vi "Acq Fetch Waveform (I16 Data Ref) - Timeout fix.vi"(0 "session in":refnum<class "Digitizer Control.lvclass">, 2 "elements to read":u32, 5 "error in (no error)":errorcluster, 7 "timeout (ms)":i32=5000, 8 "channel index":i32, 9 "clear time out error? (F)":bool) -> (13 "timed out?":bool, 14 "session out":refnum<class "Digitizer Control.lvclass">, 15 "sample data":refnum<data-value>, 16 "elements in region":u32, 17 "elements remaining":u32, 19 "error out":errorcluster)   [LabVIEW 2021, in "Digitizer Control.lvclass"]
doc: "This VI returns a reference to the host DMA buffer part containing the requested amount of acquired sample data as an array of I16s. Use the <B>Acq Configure Channel.vi</B> to configure the channel parameters, the <B>Acq Configure Transfer.vi</B> to configure the waveform transfer, and the <B>Acq Configure Start Trigger.vi</B> to configure the start trigger, then use the <B>Acq Initiate.vi</B> to initiate the acquisition. After the acquisition is initiated, use this VI to fetch the acquired sample data. Use the <B>Acq Get Status.vi</B> to check the acquisition status and the <B>Acq Stop.vi</B> to stop an acquisition.\n\nInputs:\n\n<B>session in</B>: The device session.\n\n<B>channel index</B>: The index of the channel to read.\n\n<B>elements to read</B>: The desired number of I16 elements the referenced array should contain. The actual number of elements is returned on the <B>elements in region</B> output.\n\n<B>timeout</B>: The maximum amount of time, in milliseconds, this VI is allowed to wait for the requested number of elements to become available.\n\n<B>clear time out error?</B>: If this input is true, then the <B>error out</B> output does not return the time out error.\n\nOutputs:\n\n<B>session out</B>: The device session passed on the <B>session in</B> input.\n\n<B>sample data</B>: Reference to an array of I16s containing the acquired sample data. The samples are using fixed point representation: the size of a sample is <B>sample size (bits)</B> bits. The bits of the samples are placed in the I16 elements with LSB first bit packing. To convert the returned I16 array to samples scaled to Volts: unpack the samples then multiply the samples by <B>sample scale factor</B> * 2^-( <B>sample size (bits)</B> ), where <B>sample scale factor</B> is returned by the <B>Acq Configure Channel.vi</B>, while <B>sample size (bits)</B> is returned by the <B>Acq Configure Transfer.vi</B>. The size of the array referenced by this output is returned on the <B>elements in region</B> output. NOTE: The returned data value reference must be deleted after it is no longer needed.\n\n<B>elements in region</B>: The number of I16 elements available in the array referenced by the <B>sample data</B> output.\n\n<B>elements remaining</B>: The number of additional elements remaining in the host DMA buffer that are available for reading.\n\n<B>timed out?</B>: A true on this output indicates that the fetch operation timed out.\n\nNotes:\n\nDo not mix the different Acq Fetch Waveform VIs. Once this VI is called on a channel, use only this VI to fetch the acquired samples on that channel. If you want to use another fetch VI, then it is recommended to reconfigure the transfer first using the <B>Acq Configure Transfer.vi</B>."
uses:
  Digitizer Control.lvclass
  Digitizer Control.lvclass/Digitizer Control.ctl
  <vilib>/rvi/errors/niLvFpgaAdjustHostInterfaceError.vi
  <vilib>/rvi/interface/nirviMethod/nirviMethod.xnode
  <vilib>/ErrorRing/Error Ring.xnode
  <vilib>/FPGAPlugInAG/Dynamic/niLvFpga_AcquireReadRegionFifo_Dynamic.vi
  <vilib>/rvi/errors/niLvFpgaMergeErrorWithErrorCode.vi
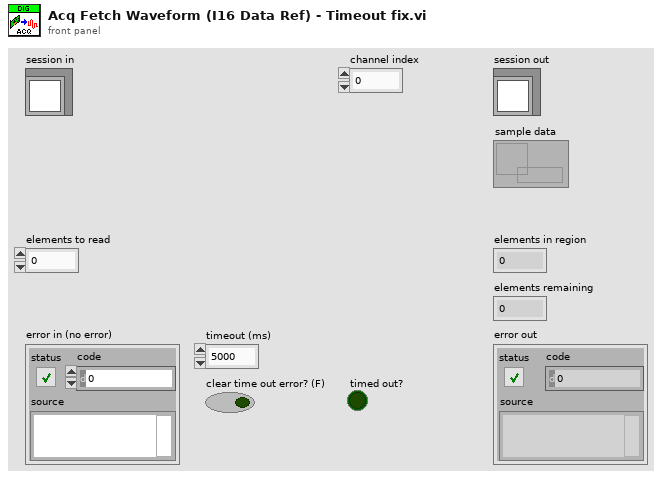
[diagram p1: front panel]
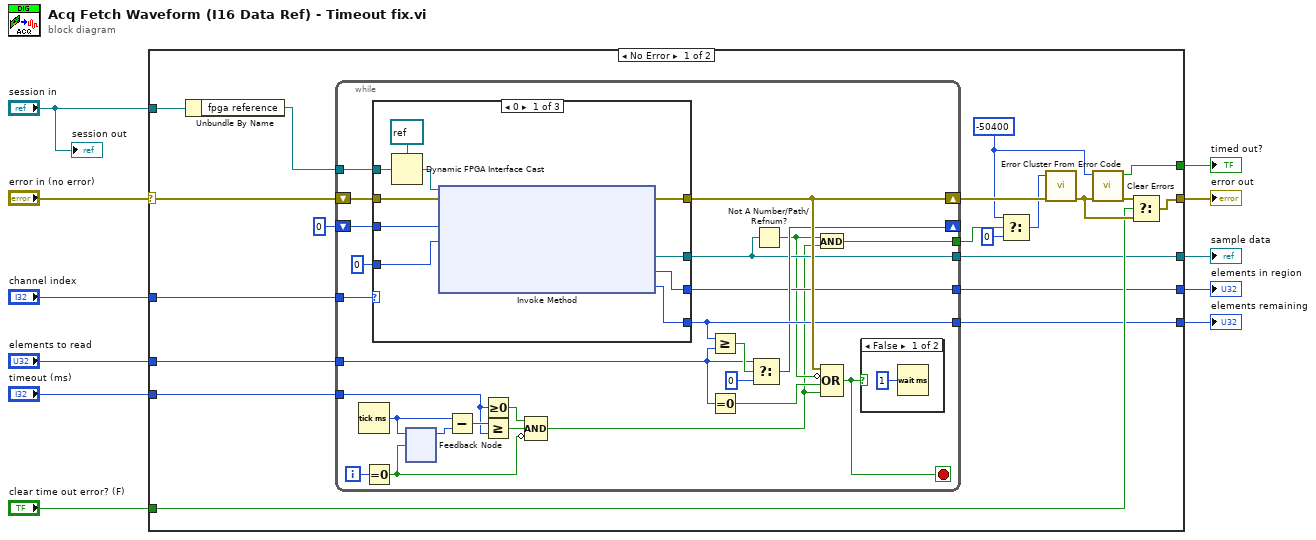
[diagram p0: block diagram]
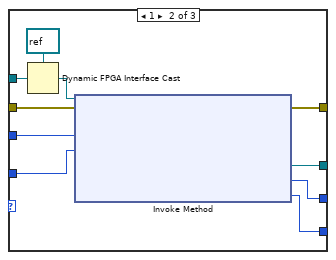
[diagram p3: hidden frame]
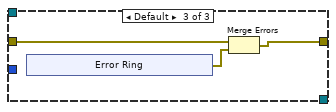
[diagram p4: hidden frame]
diagram:
  n1 = case shown="No Error" "error in (no error)" {
    selector: "error in (no error)" -> [w22 w87]
    tunnel: "elements to read" -> [w17 _]
    tunnel: [w30 w87] -> w4
    tunnel: "timeout (ms)" -> [w16 _]
    tunnel: "session in" -> [w26 _]
    tunnel: [w24 _] -> w8
    tunnel: [w25 _] -> w6
    tunnel: [w23 _] -> w5
    tunnel: "clear time out error? (F)" -> [w27 _]
    tunnel: [w20 _] -> w2
    tunnel: "channel index" -> [w19 _]
    frame No Error {
      w14 = -50400 ("specific error code to clear (0: all)")
      n2 = Unbundle By Name(w26) -> ("fpga reference"=w21:refnum<k20>)
      n3 = while {
        tunnel: [w38] -> w25
        tunnel: [w50] -> w24
        tunnel: [w39] -> w23
        tunnel: w21 -> [w54]
        tunnel: w19 -> [w53]
        shift-right: [w57] -> w29
        shift-left: w22 -> [w55]
        shift-right: [w47] -> _
        shift-left: u32 0 -> [w52]
        tunnel: w17 -> [w37]
        tunnel: w16 -> [w41]
        tunnel: [w32] -> w15
        i -> [w36]
        stop <- w35 stop-if-true
        n4 = Tick Count (ms)() -> (millisecond timer value=w46:u32)
        n5 = Equal To 0?(x=w36) -> (x = 0?=w42:bool)
        n6 = case shown="0" w53 {
          tunnel: 0 ("timeout (ms)") -> [w68 w78 _]
          tunnel: w52 -> [w65 w75 _]
          tunnel: [w64 w74 _] -> w38
          tunnel: [w63 w73 _] -> w50
          tunnel: [w62 w72 _] -> w39
          tunnel: w55 -> [w61 w71 w80]
          tunnel: w54 -> [w60 w70 _]
          tunnel: [w59 w69 w79] -> w57
          frame 0 {
            n7 = Dynamic FPGA Interface Cast(Session In=refnum<k20> refnum ("Type"), Type=w60) -> (Session Out=w67:refnum<k20>)
            n8 = xnode "Invoke Method"("FPGA VI Reference In"=w67, "error in"=w61, "Number of Elements"=w65, "Timeout (ms)"=w68) -> ("error out"=w59:errorcluster, "Read Region Reference"=w64:refnum<data-value>, "Elements In Region"=w62:u32, "Elements Remaining"=w63:u32)  [unwired: 1 out]
          }
          frame 1 {
            n9 = Dynamic FPGA Interface Cast(Session In=refnum<k20> refnum ("Type"), Type=w70) -> (Session Out=w77:refnum<k20>)
            n10 = xnode "Invoke Method"("FPGA VI Reference In"=w77, "error in"=w71, "Number of Elements"=w75, "Timeout (ms)"=w78) -> ("error out"=w69:errorcluster, "Read Region Reference"=w74:refnum<data-value>, "Elements In Region"=w72:u32, "Elements Remaining"=w73:u32)  [unwired: 1 out]
          }
          frame Default {
            n11 = xnode "Error Ring"() -> ("error out"=w81:errorcluster)
            n12 = Merge Errors(w80, w81) -> (w79:errorcluster)
          }
        }
        n13 = feedback-in #1(w46, w42) -> ()
        n14 = feedback #1() -> (w45:u32)  [unwired: 1 in]
        n15 = Subtract(x=w46, y=w45) -> (x-y=w44:u32)
        n16 = Greater Or Equal To 0?(x=w41) -> (x >= 0?=w40:bool)
        n17 = Greater Or Equal?(x=w44, y=w41) -> (x >= y?=w43:bool)
        n18 = Compound Arithmetic op=AND(w40, w43, invert w42) -> (w33:bool)
        n19 = Greater Or Equal?(x=w50, y=w37) -> (x >= y?=w49:bool)
        n20 = Equal To 0?(x=w37) -> (x = 0?=w56:bool)
        n21 = Select(t=w37, s=w49, f=u32 0) -> (s? t:f=w47:u32)
        n22 = Not A Number/Path/Refnum?(number/path/refnum=w38) -> (NaN/Path/Refnum?=w34:bool)
        n23 = And(x=w34, y=w33) -> (x .and. y?=w32:bool)
        n24 = Compound Arithmetic op=OR(w57, invert w34, w56, w33) -> (w35:bool)
        n25 = case shown="False" w35 {
          frame False {
            n26 = Wait (ms)(milliseconds to wait=u32 1) -> ()  [unwired: 1 out]
          }
          frame True {
          }
        }
      }
      n27 = Select(t=w14, s=w15, f=0) -> (s? t:f=w12:i32)
      n28 = call <vilib>:"Error Cluster From Error Code.vi"("error in (no error)"=w29, "error code (0)"=w12) -> ("error out"=w28:errorcluster)  [unwired: 7 in]
      n29 = call <vilib>:"Clear Errors.vi"("error in (no error)"=w28, "specific error code to clear (0: all)"=w14) -> ("error out"=w31:errorcluster, "specific error cleared?"=w20:bool)  [unwired: 4 in]
      n30 = Select(t=w31, s=w27, f=w28) -> (s? t:f=w30:errorcluster)
    }
    frame Error {
    }
  }
  "elements remaining" <- w8
  "sample data" <- w6
  "elements in region" <- w5
  "error out" <- w4
  "timed out?" <- w2
  "session out" <- "session in"
